vi "LVSWrt_Rd_Trm_noopen.vi"(7 "error in":errorcluster, 8 "WriteBuf":string="?", 10 "Comm Handle":u32) -> (0 "error out":errorcluster, 1 "string read":string, 3 "Comm Handle Out":u32)   [LabVIEW 2017]
uses:
  instr.lib/lvserial/lvserial.lvlib
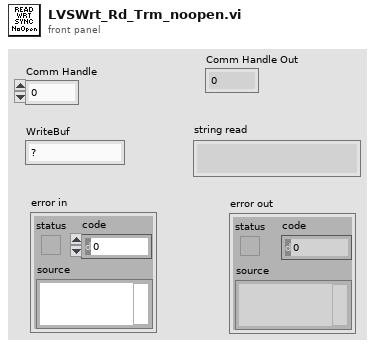
[diagram p1: front panel]
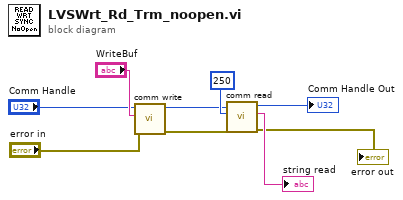
[diagram p0: block diagram]
diagram:
  n1 = call "comm write.vi"("error in (no error)"="error in", "string to write"="WriteBuf", "Comm Handle"="Comm Handle") -> ("error out"=w5:errorcluster, "dup Comm Handle"=w6:u32)  [unwired: 6 in, 1 out]
  n2 = call "comm read.vi"("error in (no error)"=w5, "requested byte count"=u32 250, "Comm Handle"=w6) -> ("error out"=→"error out":errorcluster, "string read"=→"string read":string, "dup Comm Handle"=→"Comm Handle Out":u32)  [unwired: 5 in, 1 out]
